vi "Send State Updates.vi"(8 "error in (no error)":errorcluster, 11 "Engine Data in":T1) -> (0 "error out":errorcluster, 3 "Engine Data out":T1)   [LabVIEW 2017, in "Routing and Faulting Engine.lvlib"]
uses:
  Routing and Faulting Engine.lvlib
  Engine Data.ctl
  Includes/CDMessaging.lvlibp/Producer/Abstract Producer/Abstract Producer.lvclass
  Shared/Compiled.Settings.ctl
  Shared/Communication Configuration.ctl
  Shared/Routing and Faulting Configuration.ctl
  Shared/Routing Channel Configuration.ctl
  Shared/Value-Connections Map.ctl
  Shared/Connection.ctl
  Shared/Alias Mapping.ctl
  Shared/FIFO Indices.ctl
  Device Inputs.ctl
  Device Outputs.ctl
  Shared/Routing and Faulting Shared.lvlib
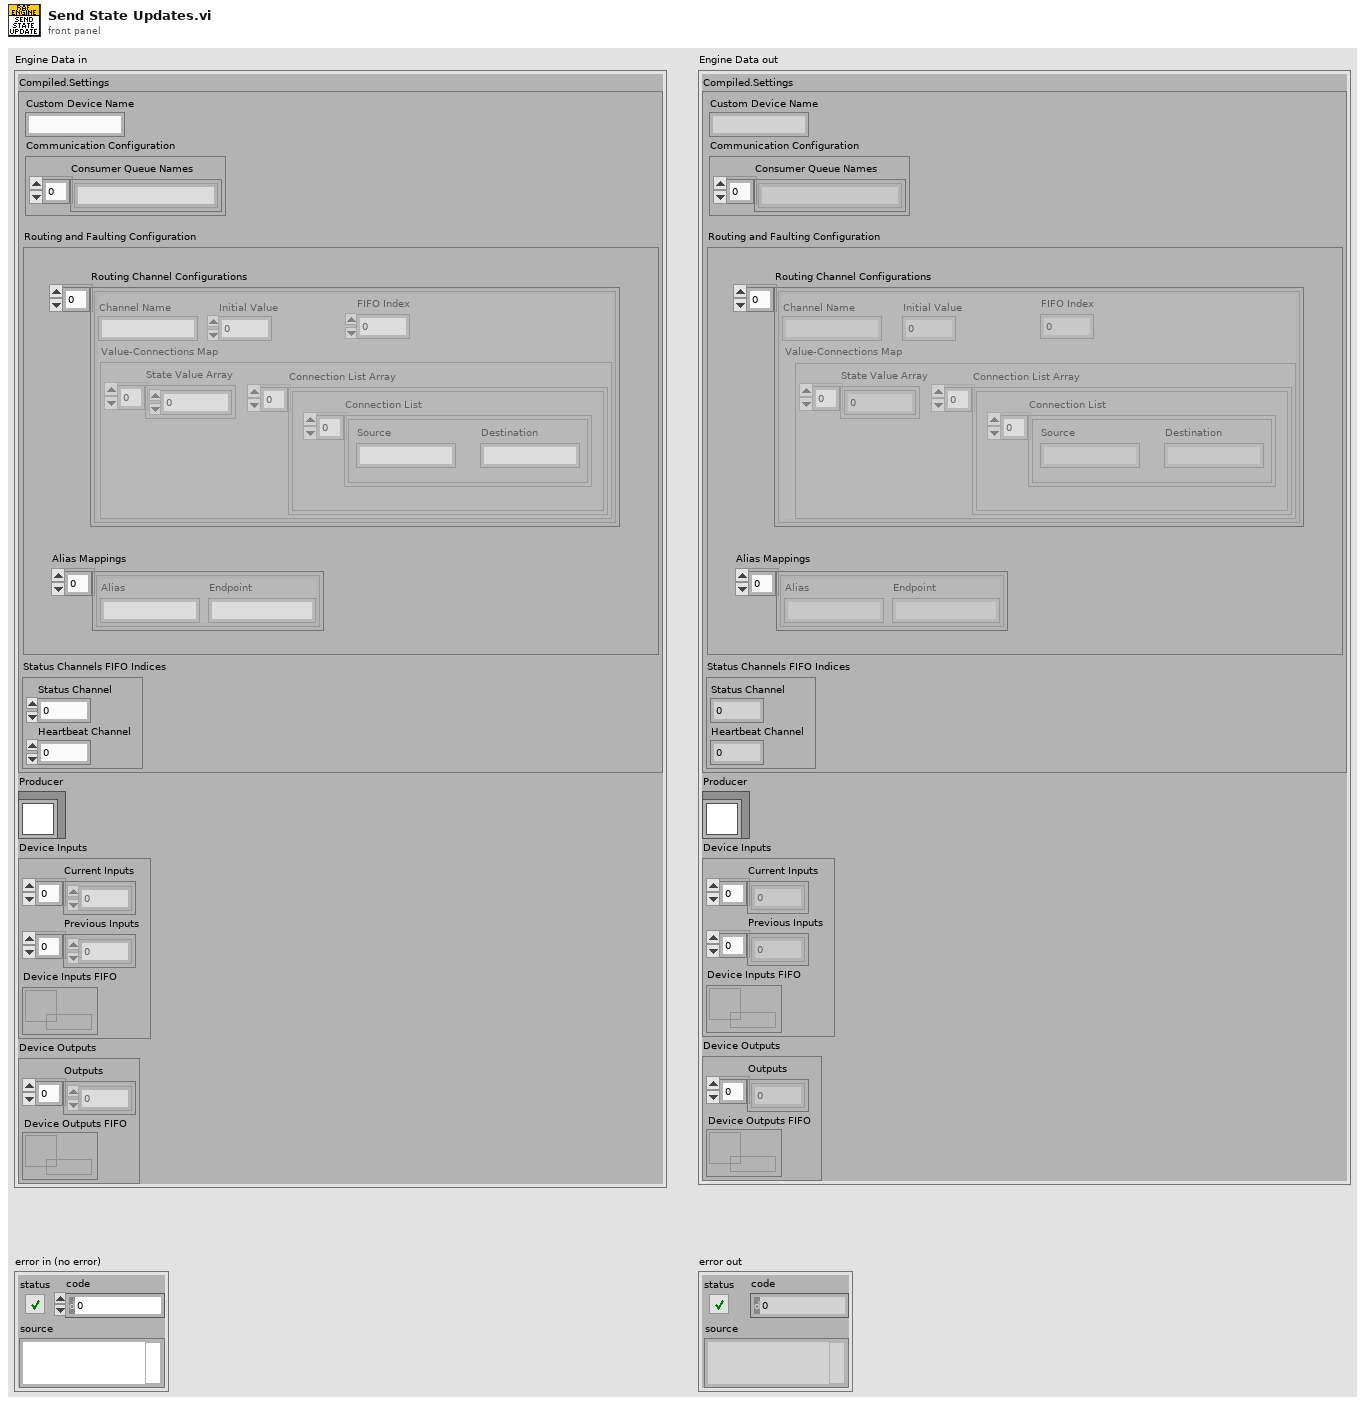
[diagram p1: front panel]
types:
  T1 = typedef "Routing and Faulting Engine.lvlib/Engine Data.ctl" = cluster{"Compiled.Settings":T2, "Producer":refnum<class "Abstract Producer.lvclass">, "Device Inputs":T10, "Device Outputs":T11}
  T2 = typedef "Routing and Faulting Shared.lvlib/Compiled.Settings.ctl" = cluster{"Custom Device Name":string, "Communication Configuration":T3, "Routing and Faulting Configuration":T4, "Status Channels FIFO Indices":T9}
  T3 = typedef "Routing and Faulting Shared.lvlib/Communication Configuration.ctl" = cluster{"Consumer Queue Names":string[]}
  T4 = typedef "Routing and Faulting Shared.lvlib/Routing and Faulting Configuration.ctl" = cluster{"Routing Channel Configurations":T5[], "Alias Mappings":T8[]}
  T5 = typedef "Routing and Faulting Shared.lvlib/Routing Channel Configuration.ctl" = cluster{"Channel Name":string, "Initial Value":dbl, "FIFO Index":i32, "Value-Connections Map":T6}
  T6 = typedef "Routing and Faulting Shared.lvlib/Value-Connections Map.ctl" = cluster{"State Value Array":i32[], "Connection List Array":cluster{"Connection List":T7[]}[]}
  T7 = typedef "Routing and Faulting Shared.lvlib/Connection.ctl" = cluster{"Source":string, "Destination":string}
  T8 = typedef "Routing and Faulting Shared.lvlib/Alias Mapping.ctl" = cluster{"Alias":string, "Endpoint":string}
  T9 = typedef "Routing and Faulting Shared.lvlib/FIFO Indices.ctl" = cluster{"Status Channel":i32, "Heartbeat Channel":i32}
  T10 = typedef "Routing and Faulting Engine.lvlib/Device Inputs.ctl" = cluster{"Current Inputs":dbl[], "Previous Inputs":dbl[], "Device Inputs FIFO":refnum<k33>}
  T11 = typedef "Routing and Faulting Engine.lvlib/Device Outputs.ctl" = cluster{"Outputs":dbl[], "Device Outputs FIFO":refnum<k33>}
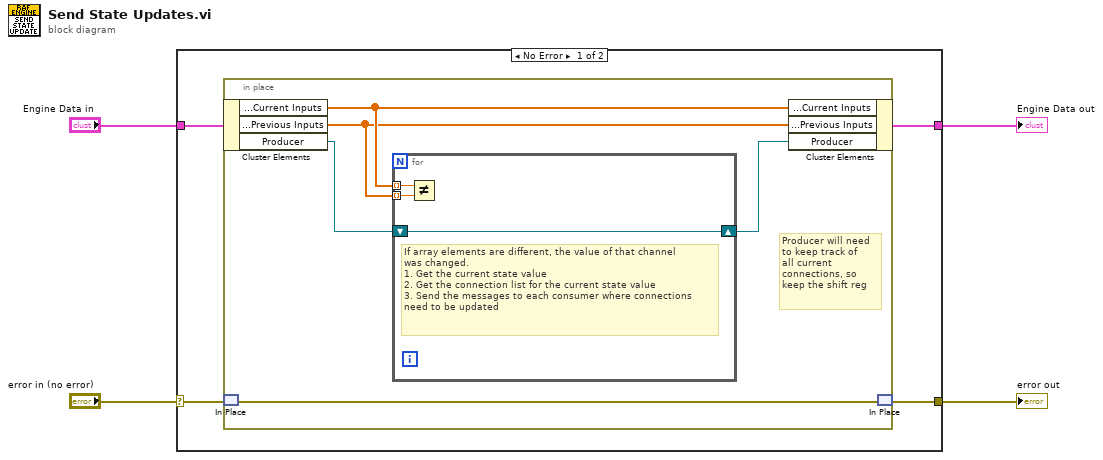
[diagram p0: block diagram]
diagram:
  n1 = case shown="No Error" "error in (no error)" {
    selector: "error in (no error)" -> [w8 w18]
    tunnel: "Engine Data in" -> [w6 w17]
    tunnel: [w7 w18] -> w2
    tunnel: [w5 w17] -> w1
    frame No Error {
      n2 = in-place {
        # "Producer will need\nto keep track of\nall current\nconnections, so\nkeep the shift reg"
        n3 = in-place-cluster #1(w6) -> ("Device Inputs.Current Inputs"=w11:dbl[], "Device Inputs.Previous Inputs"=w10:dbl[], "Producer"=w12:refnum<class "Abstract Producer.lvclass">)
        n4 = in-place-match #2(w8) -> (w13:errorcluster)
        n5 = for {
          tunnel: w10 -> [w15] mode=indexing
          tunnel: w11 -> [w16] mode=indexing
          shift-right: [w14] -> w9
          shift-left: w12 -> [w14]
          # "If array elements are different, the value of that channel\nwas changed.\n1. Get the current state value\n2. Get the connection list for the current state value\n3. Send the messages to each consumer where connections\nneed to be updated"
          n6 = Not Equal?(x=w16, y=w15) -> ()  [unwired: 1 out]
        }
        n7 = in-place-cluster #1("Device Inputs.Current Inputs"=w11, "Device Inputs.Previous Inputs"=w10, "Producer"=w9) -> (w5:T1)
        n8 = in-place-match #2(w13) -> (w7:errorcluster)
      }
    }
    frame Error {
    }
  }
  "Engine Data out" <- w1
  "error out" <- w2
